vi "ULTIMO ELEMENTO.vi"(1 "Array":dbl[](array[numeric])) -> (5 "Mean Value 2":dbl)   [LabVIEW 2009]
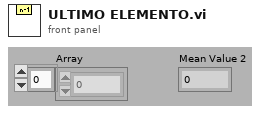
[diagram p1: front panel]
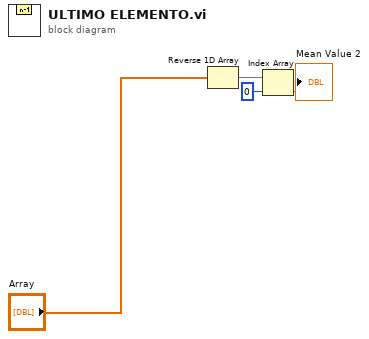
[diagram p0: block diagram]
diagram:
  n1 = Reverse 1D Array(array="Array") -> (reversed array=w1:dbl[])
  n2 = Index Array(array=w1, index=0) -> (element=→"Mean Value 2":dbl)
